vi "Write Active Logs.vi"(8 "error in (no error)":errorcluster, 10 "Logs":T1, 11 "ActiveModulesContainer in":refnum<class "ActiveModulesContainer.lvclass">) -> (0 "error out":errorcluster, 3 "ActiveModulesContainer out":refnum<class "ActiveModulesContainer.lvclass">)   [LabVIEW 2019, in "ActiveModulesContainer.lvlib" / "ActiveModulesContainer.lvclass"]
uses:
  ActiveModulesContainer.lvclass
  <vilib>/ActorFramework/Message Enqueuer/Message Enqueuer.lvclass
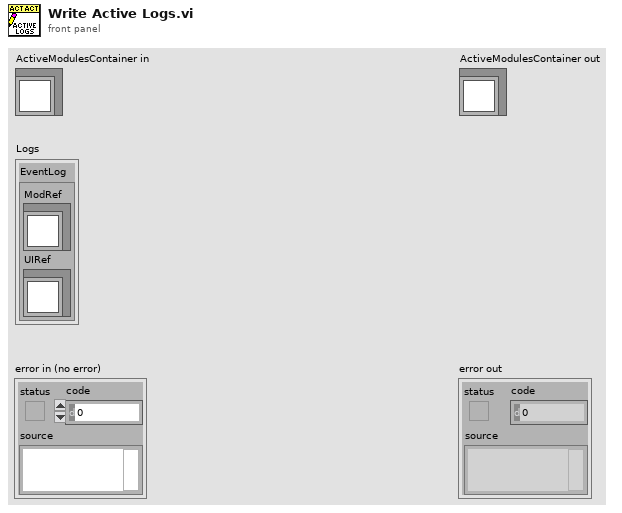
[diagram p1: front panel]
types:
  T1 = cluster{"EventLog":cluster{"ModRef":refnum<class "Message Enqueuer.lvclass">, "UIRef":refnum<class "Message Enqueuer.lvclass">}}
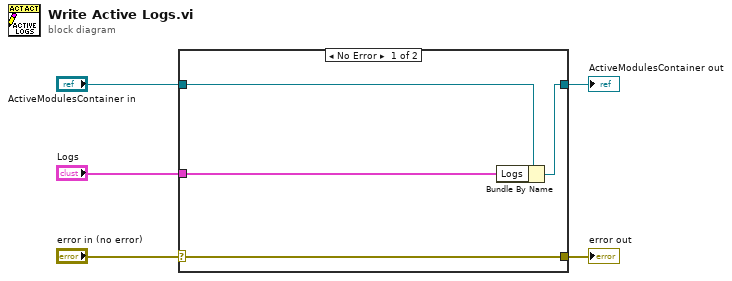
[diagram p0: block diagram]
diagram:
  n1 = case shown="No Error" "error in (no error)" {
    selector: "error in (no error)" -> [w9 w10]
    tunnel: [w9 w10] -> w4
    tunnel: [w7 w11] -> w2
    tunnel: "ActiveModulesContainer in" -> [w8 w11]
    tunnel: "Logs" -> [w6 _]
    frame No Error {
      n2 = Bundle By Name(cluster=w8, "Logs"=w6) -> (w7:refnum<class "ActiveModulesContainer.lvclass">)
    }
    frame Error {
    }
  }
  "error out" <- w4
  "ActiveModulesContainer out" <- w2
